vi "compare.vi"(1 "isOk?":refnum<vi>, 2 "IP":string) -> (0 "isOk?":bool)   [LabVIEW 2021]
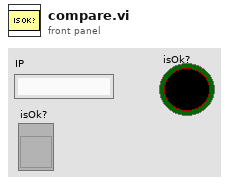
[diagram p1: front panel]
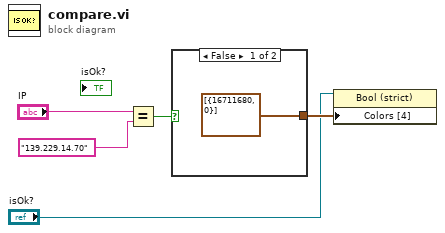
[diagram p0: block diagram]
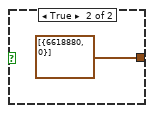
[diagram p2: hidden frame]
diagram:
  n1 = Equal?(x="IP", y="139.229.14.70") -> (x = y?=w3:bool)
  n2 = case shown="False" w3 {
    tunnel: [cluster{u32, u32}[] [{16711680, 0}] ("Colors [4]") cluster{u32, u32}[] [{6618880, 0}] ("Colors [4]")] -> w2
    frame False {
    }
    frame True {
    }
  }
  n3 = property on="Property Node" class="Bool (strict)"(reference="isOk?", "Colors [4]"=w2) -> ()  [unwired: 1 in, 2 out]
